vi "Database.Cache.Identify.vi"(8 "error in (no error)":errorcluster, 9 "Variant":string, 10 "SystemName":string, 11 "DB Handle in":i32) -> (0 "error out":errorcluster, 2 "SytemID":T1, 3 "DB Handle out":i32)   [LabVIEW 2016]
uses:
  ProdaNG/Controls/ProdaNG.Identification.ctl
  Cache/Cache.SystemID.Fglb.Action.ctl
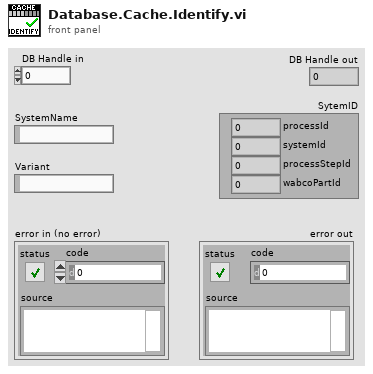
[diagram p1: front panel]
types:
  T1 = typedef "ProdaNG.Identification.ctl" = cluster{"processId":i32, "systemId":i32, "processStepId":i32, "wabcoPartId":i32}
  T2 = typedef "Cache.SystemID.Fglb.Action.ctl" = enum16{"init", "add", "get"}
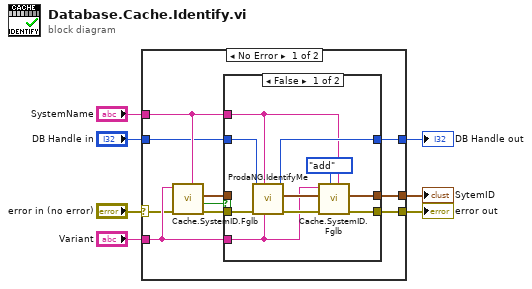
[diagram p0: block diagram]
diagram:
  n1 = case shown="No Error" "error in (no error)" {
    selector: "error in (no error)" -> [w8 w32]
    tunnel: [w17 w32] -> w7
    tunnel: [w16 w31] -> w6
    tunnel: "Variant" -> [w15 _]
    tunnel: "SystemName" -> [w14 _]
    tunnel: "DB Handle in" -> [w13 w31]
    tunnel: [w9 _] -> w2
    frame No Error {
      n2 = call "Cache.SystemID.Fglb.vi"("Station"=w14, "error in (no error)"=w8, "Variant"=w15) -> ("error out"=w12:errorcluster, "Found"=w11:bool, "SytemID"=w10:T1)  [unwired: 6 in]
      n3 = case shown="False" w11 {
        tunnel: w13 -> [w26 w29]
        tunnel: [w25 w29] -> w16
        tunnel: [w23 w30] -> w17
        tunnel: w12 -> [w21 w30]
        tunnel: w15 -> [w20 _]
        tunnel: w14 -> [w19 _]
        tunnel: w10 -> [_ w28]
        tunnel: [w18 w28] -> w9
        frame False {
          n4 = call "ProdaNG.IdentifyMe.vi"("wabcoNumber"=w20, "systemName"=w19, "error in"=w21, "dbHandleIn"=w26) -> ("error out"=w24:errorcluster, "Identification"=w27:T1, "dbHandle"=w25:i32)  [unwired: 5 in]
          n5 = call "Cache.SystemID.Fglb.vi"("Station"=w19, "Action (get)"=Cache.SystemID.Fglb.Action."add", "error in (no error)"=w24, "SytemID"=w27, "Variant"=w20) -> ("error out"=w23:errorcluster, "SytemID"=w18:T1)  [unwired: 4 in, 1 out]
        }
        frame True {
        }
      }
    }
    frame Error {
    }
  }
  "error out" <- w7
  "DB Handle out" <- w6
  "SytemID" <- w2
